vi "Main.vi"() -> ()   [LabVIEW 2019]
uses:
  Typedefs/#enum_MasterState.ctl
  Typedefs/#cluster_GUIRefs.ctl
  ResultsViewer/ResultsViewer/ResultsViewer.lvclass
  C:/Program Files (x86)/National Instruments/LabVIEW 2019/vi.lib/ActorFramework/Actor/Actor.lvclass
  SubVIs/Application Configuration VIs/#cluster_AppConfiguration.ctl
  SubVIs/LowLevelError.vi
  <vilib>/ActorFramework/Actor/Actor.lvclass
panel:
  in  "Results Viewer":bool
  in  "POX Data History":string[](array[string])
  in  "Save?":bool caption="Save Results?"
  in  "Measure":bool
  in  "Measurement Directory":path
  in  "Stop":bool
  out "O2 Saturation":dbl(graph)
  out "Heart beat":dbl(graph)
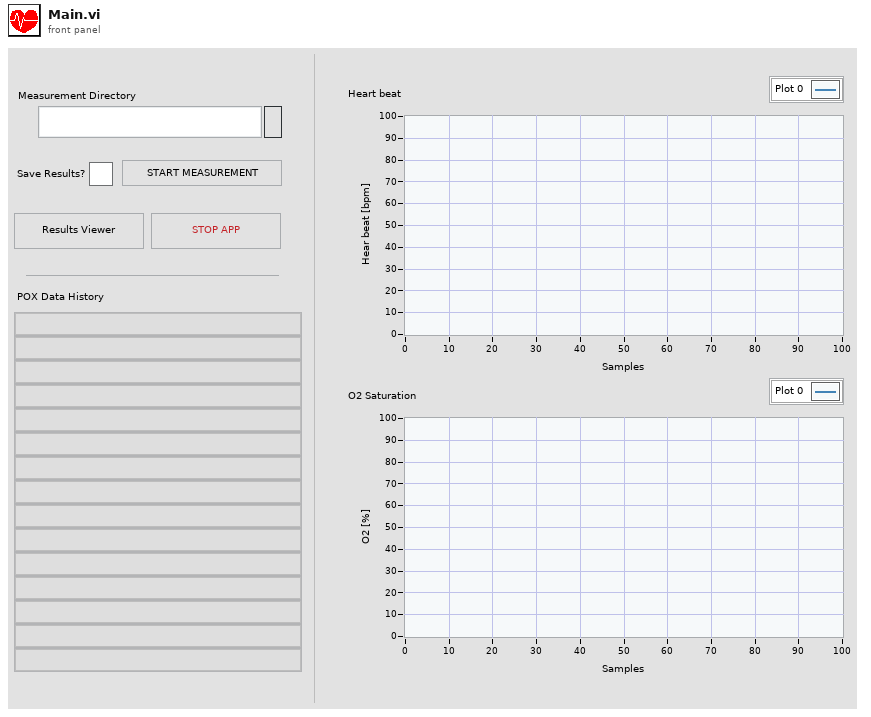
[diagram p1: front panel]
types:
  T1 = typedef "#enum_MasterState.ctl" = enum16{"Idle", "Init", "Close", "Error"}
  T2 = typedef "#cluster_ApplicationData.ctl" = cluster{"Acq Queue":refnum<queue>, "Saving Queue":refnum<queue>}
  T3 = typedef "#cluster_GUIRefs.ctl" = cluster{"Measure":refnum<vi>, "Save?":refnum<vi>, "Stop":refnum<vi>, "Measurement Dir":refnum<vi>, "Heart beat":refnum<vi>, "O2":refnum<vi>, "POX Data History":refnum<vi>}
  T4 = typedef "#cluster_AppConfiguration.ctl" = cluster{"Measurements Directory":path}
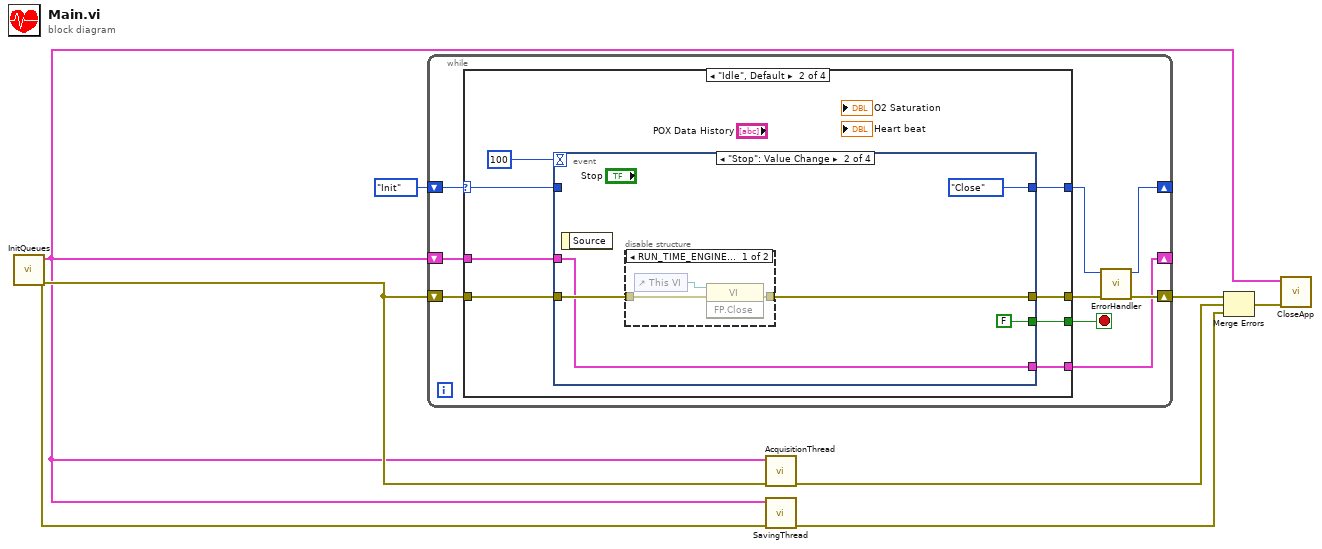
[diagram p0: block diagram]
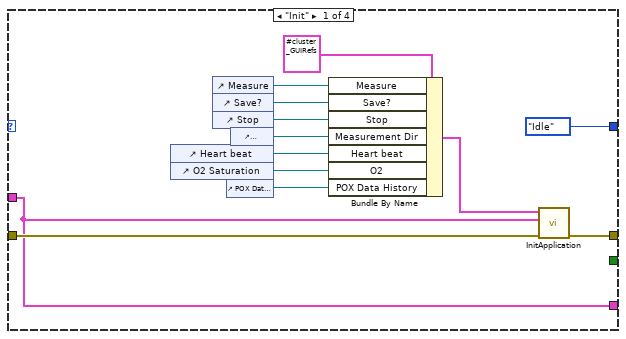
[diagram p2: hidden frame]
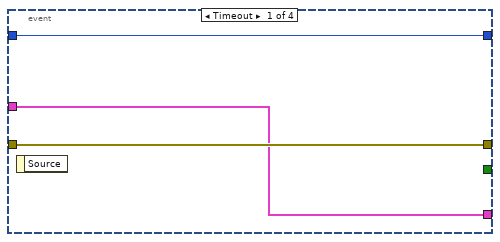
[diagram p3: hidden frame]
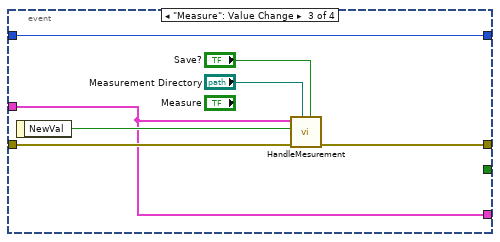
[diagram p5: hidden frame]
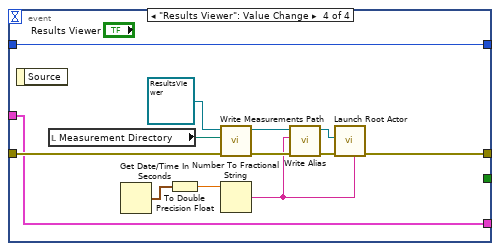
[diagram p6: hidden frame]
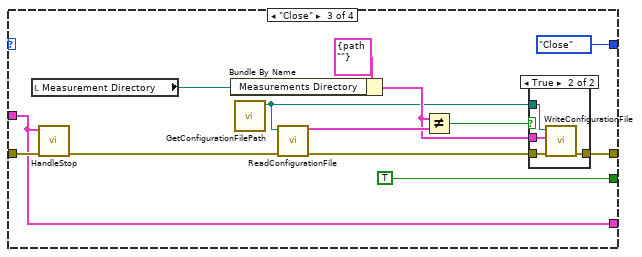
[diagram p7: hidden frame]
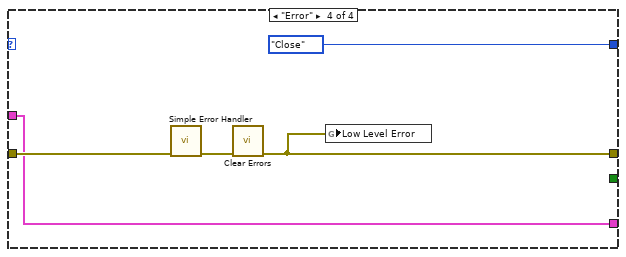
[diagram p9: hidden frame]
diagram:
  n1 = call "InitQueues.vi"() -> ("error out"=w3:errorcluster, "Application Data"=w2:T2)  [unwired: 10 in]
  n2 = while {
    shift-right: [w11] -> w7
    shift-left: w3 -> [w16]
    shift-right: [w9] -> _
    shift-left: #enum_MasterState."Init" ("Master State") -> [w13]
    shift-right: [w8] -> _
    shift-left: w2 -> [w15]
    stop <- w14 stop-if-true
    n3 = case shown="\"Idle\", Default" w13 {
      selector: w13 -> [_ w34 _ _]
      tunnel: w16 -> [w22 w37 w82 w91]
      tunnel: w15 -> [w17 w31 w70 w88]
      tunnel: [w20 w36 w76 w89] -> w12
      tunnel: [_ w35 TRUE _] -> w14
      tunnel: [#enum_MasterState."Idle" ("Master State") w33 #enum_MasterState."Close" ("Master State") #enum_MasterState."Close" ("Master State")] -> w10
      tunnel: [w17 w30 w70 w88] -> w8
      frame "Init" {
        n4 = control-ref of="Heart beat"() -> (w28:refnum<vi>)
        n5 = control-ref of="O2 Saturation"() -> (w29:refnum<vi>)
        n6 = control-ref of="Measure"() -> (w24:refnum<vi>)
        n7 = control-ref of="Save?"() -> (w25:refnum<vi>)
        n8 = control-ref of="Stop"() -> (w26:refnum<vi>)
        n9 = control-ref of="POX Data History"() -> (w18:refnum<vi>)
        n10 = control-ref of="Measurement Directory"() -> (w27:refnum<vi>)
        n11 = Bundle By Name(cluster=T3 {"Measure"=refnum, "Save?"=refnum, "Stop"=refnum, "Measurement Dir"=refnum, "Heart beat"=refnum, "O2"=refnum, "POX Data History"=refnum} ("GUI Refs"), "Measure"=w24, "Save?"=w25, "Stop"=w26, "Measurement Dir"=w27, "Heart beat"=w28, "O2"=w29, "POX Data History"=w18) -> (w21:T3)
        n12 = call "InitApplication.vi"("error in (no error)"=w22, "Application Data in"=w17, "GUI Refs"=w21) -> ("error out"=w20:errorcluster)  [unwired: 8 in]
      }
      frame "Idle", Default {
        n13 = event shown="[1] \"Stop\": Value Change" {
          selector: _ -> [_ _ _ _]
          dyn-events: _ -> [_ _ _ _]
          timeout: 100 -> [_ _ _ _]
          tunnel: w37 -> [w40 w45 w56 w69]
          tunnel: w31 -> [w38 w42 w50 w63]
          tunnel: [w40 w41 w54 w64] -> w36
          tunnel: [_ FALSE _ _] -> w35
          tunnel: w34 -> [w39 _ w51 w62]
          tunnel: [w39 #enum_MasterState."Close" ("Master State") w51 w62] -> w33
          tunnel: [w38 w42 w50 w63] -> w30
          event Timeout {
            n14 = event-data() -> ()  [unwired: 1 in, 1 out]
          }
          event "Stop": Value Change {
            n15 = event-data() -> ()  [unwired: 1 in, 1 out]
            n16 = disable-structure shown="RUN_TIME_ENGINE==True" {
              disable-tunnel: w45 -> [w48 w49]
              disable-tunnel: [w47 w49] -> w41
              frame condition #0 {
                n17 = control-ref of="This VI"() -> (w46:refnum<vi>)
                n18 = invoke class="VI" method="FP.Close"(reference=w46, error in=w48) -> (error out=w47:errorcluster)  [unwired: 1 in, 2 out]
              }
              frame condition #1 (active) {
              }
            }
          }
          event "Measure": Value Change {
            n19 = event-data() -> ("NewVal"=w55:bool)  [unwired: 1 in]
            n20 = call "HandleMesurement.vi"("Save?"="Save?", "Measurement Directory"="Measurement Directory", "error in (no error)"=w56, "Measure?"=w55, "Application Data"=w50) -> ("error out"=w54:errorcluster)  [unwired: 6 in]
          }
          event "Results Viewer": Value Change {
            n21 = event-data() -> ()  [unwired: 1 in, 1 out]
            n22 = local read "Measurement Directory"() -> (w66:path)
            n23 = Get Date/Time In Seconds() -> (seconds since 1Jan1904=w61:timestamp)
            n24 = To Double Precision Float(number=w61) -> (double precision float=w57:dbl)
            n25 = call-dynamic "Write Measurements Path.vi"("error in (no error)"=w69, "Measurements Path"=w66, "ResultsViewer in"=refnum<class "ResultsViewer.lvclass"> refnum ("ResultsViewer.lvlib:ResultsViewer.lvclass")) -> ("error out"=w68:errorcluster, "ResultsViewer out"=w65:refnum<class "ResultsViewer.lvclass">)  [unwired: 7 in]
            n26 = Number To Fractional String(number=w57) -> (F-format string=w58:string)  [unwired: 3 in]
            n27 = call-dynamic "Write Alias.vi"("error in (no error)"=w68, "Alias"=w58, "ResultsViewer in"=w65) -> ("error out"=w60:errorcluster, "ResultsViewer out"=w59:refnum<class "ResultsViewer.lvclass">)  [unwired: 7 in]
            n28 = call <vilib>:"Launch Root Actor.vi"("Debug Alias"=w58, "error in (no error)"=w60, "Actor"=w59) -> ("error out"=w64:errorcluster)  [unwired: 7 in, 1 out]
          }
        }
      }
      frame "Close" {
        n29 = local read "Measurement Directory"() -> (w74:path)
        n30 = call "HandleStop.vi"("error in (no error)"=w82, "Application Data"=w70) -> ("error out"=w79:errorcluster)  [unwired: 9 in]
        n31 = Bundle By Name(cluster=T4 {"Measurements Directory"=path ""} ("App Configuration"), "Measurements Directory"=w74) -> (w72:T4)
        n32 = call "GetConfigurationFilePath.vi"() -> ("Configuration File Path"=w71:path)  [unwired: 11 in]
        n33 = call "ReadConfigurationFile.vi"("Error in"=w79, "Configuration File Path"=w71) -> ("Error out"=w78:errorcluster, "App Configuration"=w73:T4)  [unwired: 8 in]
        n34 = Not Equal?(x=w72, y=w73) -> (x != y?=w77:bool)
        n35 = case shown="True" w77 {
          tunnel: w78 -> [w83 w87]
          tunnel: [w83 w86] -> w76
          tunnel: w72 -> [_ w85]
          tunnel: w71 -> [_ w84]
          frame False {
          }
          frame True {
            n36 = call "WriteConfigurationFile.vi"("Error in"=w87, "App Configuration"=w85, "Configuration File Path"=w84) -> ("Error out"=w86:errorcluster)  [unwired: 8 in]
          }
        }
      }
      frame "Error" {
        n37 = call <vilib>:"Simple Error Handler.vi"("error in (no error)"=w91) -> ("error out"=w90:errorcluster)  [unwired: 4 in, 4 out]
        n38 = call <vilib>:"Clear Errors.vi"("error in (no error)"=w90) -> ("error out"=w89:errorcluster)  [unwired: 5 in, 1 out]
        n39 = global write "LowLevelError.vi" "Low Level Error"(w89) -> ()
      }
    }
    n40 = call "ErrorHandler.vi"("error in (no error)"=w12, "Master State in"=w10) -> ("error out"=w11:errorcluster, "Master State out"=w9:T1)  [unwired: 8 in]
  }
  n41 = call "AcquisitionThread.vi"("error in (no error)"=w3, "Application Data"=w2) -> ("error out"=w6:errorcluster)  [unwired: 9 in]
  n42 = call "SavingThread.vi"("error in (no error)"=w3, "Application Data"=w2) -> ("error out"=w4:errorcluster)  [unwired: 9 in]
  n43 = Merge Errors(w7, w6, w4) -> (w1:errorcluster)
  n44 = call "CloseApp.vi"("error in (no error)"=w1, "Application Data"=w2) -> ()  [unwired: 9 in, 1 out]
